vi "ObtainBroadcastForRegistration.vi"(8 "error in (no error)":errorcluster) -> (0 "error out":errorcluster, 2 "OutputToFileBroadcast":T1)   [LabVIEW 2014, in "OutputToFileModule.lvlib"]
uses:
  OutputToFileModule.lvlib
  Protected/Broadcasts/clBroadcastEvents.ctl
  Private/clEventType.ctl
panel:
  # "Rename this for each module type"
  # "If you want to add other Broadcast Events, open this typedef, copy an existing event and rename it to your event name.\n\nNext create an \"arg\" typedef for the  data and put it into PublicAPI/Arguments/Broadcasts\n\nAfter that, you will need to create a new roadcast vi in Protected/Broadcast.  Look at DidInit.vi or the reportError.vi as examples."
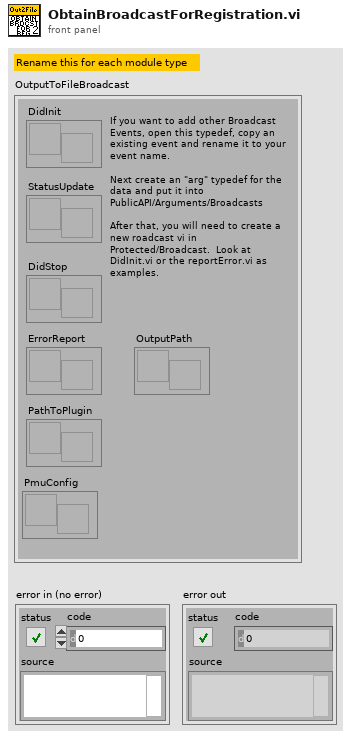
[diagram p1: front panel]
types:
  T1 = typedef "OutputToFileModule.lvlib/clBroadcastEvents.ctl" = cluster{"DidInit":refnum<user-event>, "StatusUpdate":refnum<user-event>, "ErrorReport":refnum<user-event>, "DidStop":refnum<user-event>, "PathToPlugin":refnum<user-event>, "PmuConfig":refnum<user-event>, "OutputPath":refnum<user-event>}
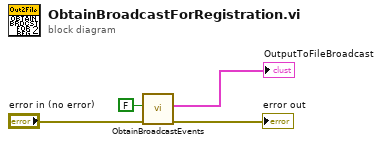
[diagram p0: block diagram]
diagram:
  n1 = call "ObtainBroadcastEvents.vi"("error in (no error)"="error in (no error)", "CreateNew? (F)"=FALSE) -> ("error out"=→"error out":errorcluster, "clBroadcastEvents"=→"OutputToFileBroadcast":T1)  [unwired: 8 in]
